vi "Remove File, If Exists.vi"(4 "error in":errorcluster, 7 "filepath":path) -> (0 "error out":errorcluster, 3 "filepath dup":path)   [LabVIEW 2010]
doc: "This function deletes a file, if it exists."
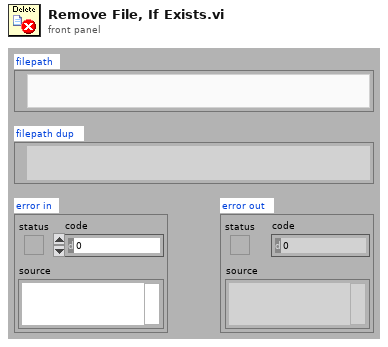
[diagram p1: front panel]
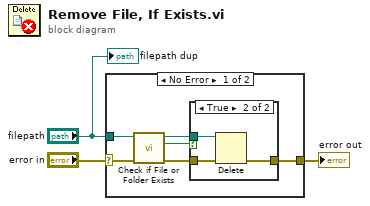
[diagram p0: block diagram]
diagram:
  n1 = case shown="No Error" "error in" {
    selector: "error in" -> [w9 w14]
    tunnel: [w8 w14] -> w2
    tunnel: "filepath" -> [w4 _]
    frame No Error {
      n2 = call <vilib>:"Check if File or Folder Exists.vi"("error in (no error)"=w9, "path"=w4) -> ("error out"=w6:errorcluster, "file or folder exists?"=w5:bool, "dup path"=w7:path)  [unwired: 7 in]
      n3 = case shown="True" w5 {
        tunnel: [w10 w13] -> w8
        tunnel: w7 -> [_ w12]
        tunnel: w6 -> [w10 w11]
        frame False {
        }
        frame True {
          n4 = Delete(path (use dialog)=w12, error in=w11) -> (error out=w13:errorcluster)  [unwired: 3 in, 2 out]
        }
      }
    }
    frame Error {
    }
  }
  "error out" <- w2
  "filepath dup" <- "filepath"
